vi "Draw.vi"(8 "error in (no error)":errorcluster, 9 "DrawPoint(Ingored If Not Wired)":T1={"X"=-1, "Y"=-1}, 10 "PictureIn":picture, 11 "reference in":refnum<class "Character.lvclass">) -> (0 "error out":errorcluster, 1 "Width":i32, 2 "PictureOut":picture, 3 "reference in":refnum<class "Character.lvclass">)   [LabVIEW 2012, in "Character.lvclass"]
uses:
  Character.lvclass
  Glyph_class/Position.ctl
  Glyph_class/Glyph.lvclass
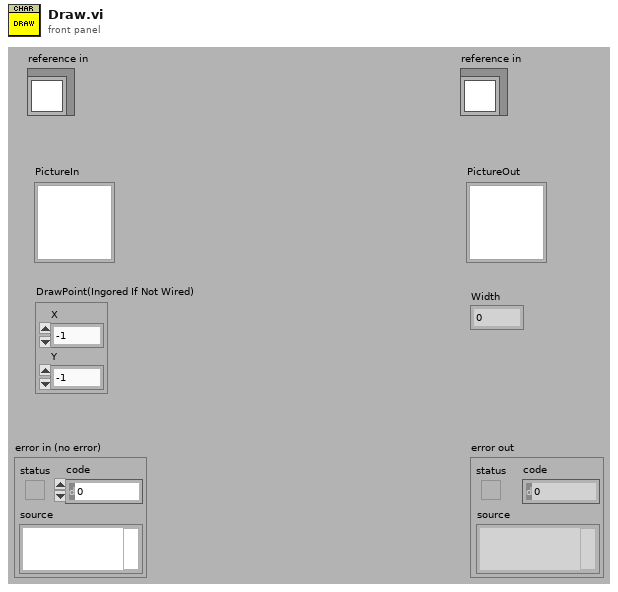
[diagram p1: front panel]
types:
  T1 = typedef "Glyph.lvclass/Position.ctl" = cluster{"X":i32, "Y":i32}
  T2 = enum16{"User-specified Font", "Application Font", "System Font", "Dialog Font"}
  T3 = typedef "Character.lvclass/ObjectAttributes.ctl" = cluster{"Font":cluster{"Font Name:":string, "Size":i16, "Strikeout?":bool, "Italic?":bool, "Underline?":bool, "Outline?":bool, "Shadow?":bool, "Bold?":bool}, "Color":u32, "Character":string}
  T4 = cluster{"Font Name:":string, "Size":i16, "Strikeout?":bool, "Italic?":bool, "Underline?":bool, "Outline?":bool, "Shadow?":bool, "Bold?":bool}
  T5 = cluster{"left":i16, "top":i16, "right":i16, "bottom":i16}
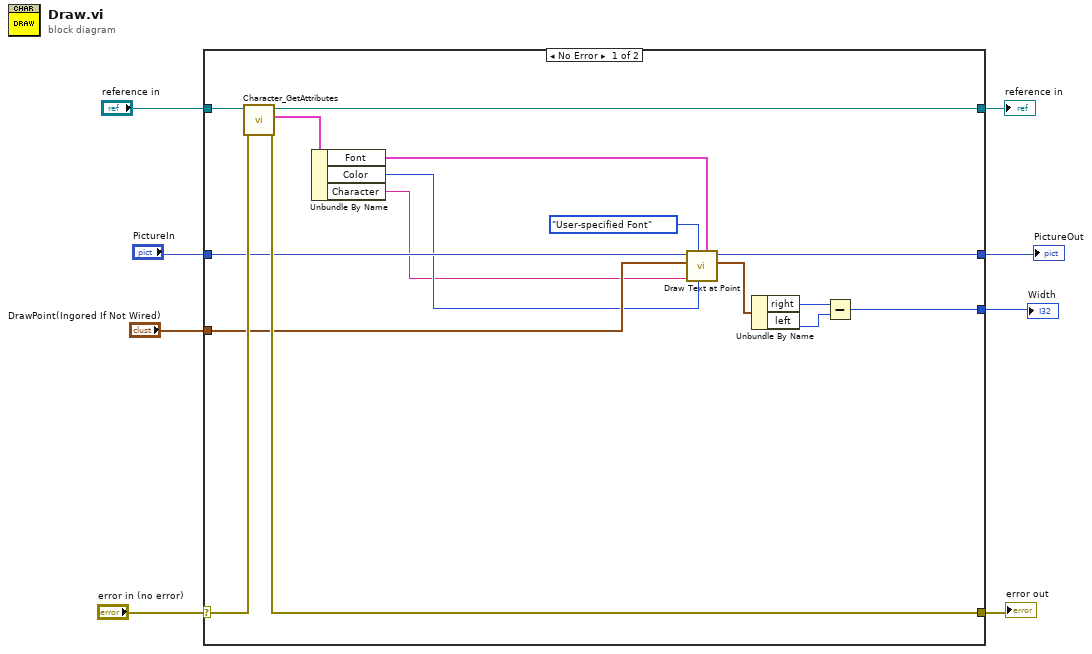
[diagram p0: block diagram]
diagram:
  n1 = case shown="No Error" "error in (no error)" {
    selector: "error in (no error)" -> [w24 w27]
    tunnel: [w22 w27] -> w7
    tunnel: [w20 w26] -> w5
    tunnel: "reference in" -> [w21 w26]
    tunnel: "PictureIn" -> [w19 w25]
    tunnel: [w18 w25] -> w3
    tunnel: "DrawPoint(Ingored If Not Wired)" -> [w17 _]
    tunnel: [w9 _] -> w1
    frame No Error {
      n2 = call "Character_GetAttributes.vi"("error in (no error)"=w24, "reference in"=w21) -> ("error out"=w22:errorcluster, "Data"=w23:T3, "reference out"=w20:refnum<class "Character.lvclass">)  [unwired: 6 in, 1 out]
      n3 = Unbundle By Name(w23) -> ("Font"=w15:T4, "Color"=w14:u32, "Character"=w12:string)
      n4 = call <vilib>:"Draw Text at Point.vi"("[user-specified font]"=w15, "text color(black)"=w14, "desired font(Application)"=T2."User-specified Font", "text"=w12, "origin"=w17, "picture"=w19) -> ("text rect"=w13:T5, "new picture"=w18:picture)  [unwired: 4 in]
      n5 = Unbundle By Name(w13) -> ("right"=w11:i16, "left"=w10:i16)
      n6 = Subtract(x=w11, y=w10) -> (x-y=w9:i16)
    }
    frame Error {
    }
  }
  "error out" <- w7
  "reference in" <- w5
  "PictureOut" <- w3
  "Width" <- w1
